vi "ROI entry screen-Update ROI and save to ROI file.vi"(8 "error in (no error)":errorcluster, 11 "Experiment folder path":path) -> (0 "Error Out":errorcluster, 2 "XYZ_Coordinates":T1[](array[typedef]) {"Apparent Frame Size" format="%#_6f"; "Original FOV (um)" format="%#_6f"; "Pixels per miniscan" format="%#_6f"; "Dwell Time per pixel" format="%#_6f"; "Resolution" format="%#_6f"; "ROI group ID" format="%#_6f"; "Laser Power (%)" format="%#_6f"; "Zoom" format="%#_6f"; "Frame Size" format="%#_6f"; "Number of lines" format="%#_6f"; "Composite ID" format="%#_6f"; "Angle (deg)" format="%#_6f"; "ROI Time (ns)" format="%#_6f"; "ROI ID" format="%#_6f"; "Pixels in ROI" format="%#_6f"; "ROI index" format="%#_6f"; "Z stop" format="%#_6f"; "Y stop" format="%#_6f"; "X stop" format="%#_6f"; "Z start" format="%#_6f"; "X start" format="%#_6f"; "Y start" format="%#_6f"})   [LabVIEW 2020]
uses:
  Visualisation/Functional Imaging Viewer/Typedefs/ROI parameters data type.ctl
  Typedefs/ROI management FG states.ctl
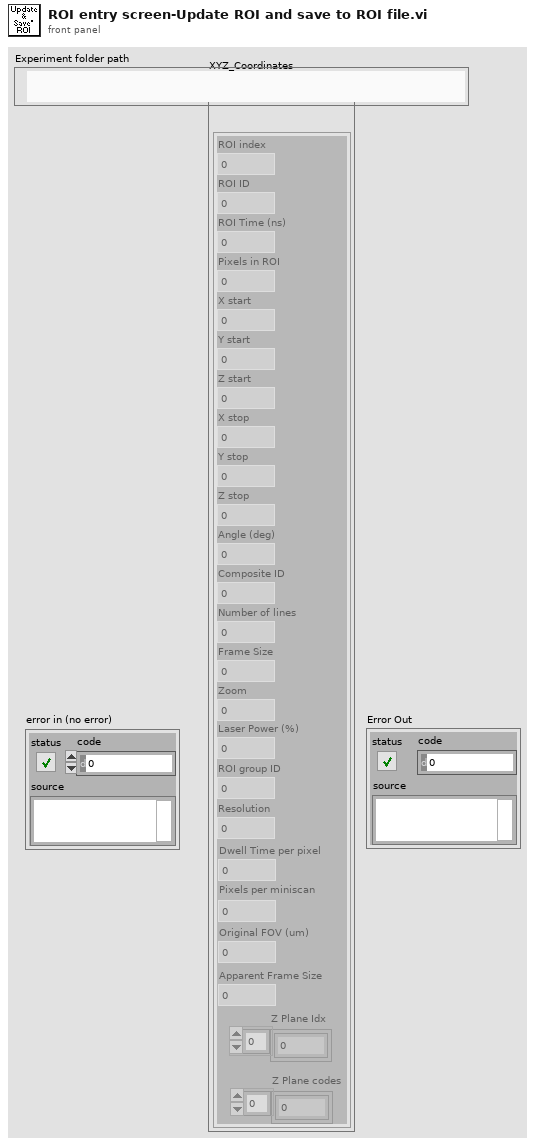
[diagram p1: front panel]
types:
  T1 = typedef "ROI parameters data type.ctl" = cluster{"ROI index":dbl, "ROI ID":dbl, "ROI Time (ns)":dbl, "Pixels in ROI":dbl, "X start":dbl, "Y start":dbl, "Z start":dbl, "X stop":dbl, "Y stop":dbl, "Z stop":dbl, "Angle (deg)":dbl, "Composite ID":dbl, "Number of lines":dbl, "Frame Size":dbl, "Zoom":dbl, "Laser Power (%)":dbl, "ROI group ID":dbl, "Resolution":dbl, "Dwell Time per pixel":dbl, "Pixels per miniscan":dbl, "Original FOV (um)":dbl, "Apparent Frame Size":dbl, "Z Plane Idx":i32[], "Z Plane codes":i32[]}
  T2 = typedef "ROI management FG states.ctl" = enum16{"Read", "Write", "Write-from dataset", "Clear Last", "Clear All", "Delete ROI", "Update ROIs time", "Reload last ROI set", "Modify ROI Parameters", "Offset all ROI", "Offset visible ROI", "Modify Dwell Time", "Modify Laser Power"}
  T3 = cluster{"XYZ Coordinates":T1[], "Norm coordinates":T1[]}
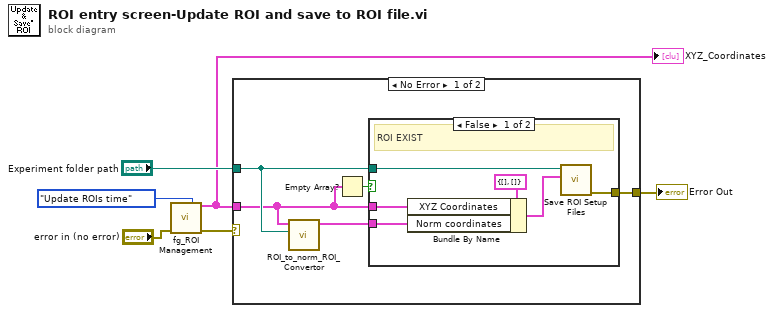
[diagram p0: block diagram]
diagram:
  n1 = call "fg_ROI Management.vi"("Function"=ROI_management_FG_states."Update ROIs time", "error in (no error)"="error in (no error)") -> ("ROI Setup"=w4:T1[], "error out"=w2:errorcluster)  [unwired: 7 in, 5 out]
  "XYZ_Coordinates" <- w4
  n2 = case shown="No Error" w2 {
    selector: w2 -> [_ w18]
    tunnel: "Experiment folder path" -> [w11 _]
    tunnel: w4 -> [w8 _]
    tunnel: [w7 w18] -> w3
    frame No Error {
      n3 = call "ROI_to_norm_ROI_Convertor.vi"("Experiment folder path"=w11, "XYZ Coordinates"=w8) -> ("norm_XYZ_Coordinates"=w10:T1[])  [unwired: 9 in]
      n4 = Empty Array?(array=w8) -> (empty?=w9:bool)
      n5 = case shown="False" w9 {
        tunnel: w8 -> [w17 _]
        tunnel: w11 -> [w14 _]
        tunnel: w10 -> [w13 _]
        tunnel: [w12 _] -> w7
        frame False {
          # "ROI EXIST"
          n6 = Bundle By Name(cluster=T3 {"XYZ Coordinates"=[], "Norm coordinates"=[]} ("ROI_Information_Cluster"), "XYZ Coordinates"=w17, "Norm coordinates"=w13) -> (w15:T3)
          n7 = call "Save ROI Setup Files.vi"("ROI_Information_Cluster"=w15, "Experiment data folder path"=w14) -> ("Error Out"=w12:errorcluster)  [unwired: 9 in]
        }
        frame True {
          # "NO ROI!"
        }
      }
    }
    frame Error {
    }
  }
  "Error Out" <- w3
